vi "map.vi"() -> ()   [LabVIEW 2024]
uses:
  C:/Program Files (x86)/National Instruments/LabVIEW 2024/examples/Design Patterns/Queued Message Handler/support/QMH Fundamentals - Message Cluster.ctl
  <extravilib>/ChannelInstances/Lossy Stream-c(i32)/Read With Abort.vi
  <extravilib>/ChannelInstances/Lossy Stream-c(u16)/Write With Abort.vi
  <extravilib>/ChannelInstances/Lossy Stream-c(u16)/Read With Abort.vi
  <extravilib>/ChannelInstances/Lossy Stream-c(i32)/Write With Abort.vi
  <extravilib>/ChannelInstances/Lossy Stream-c(i32)/EndpointRead.vi
  <extravilib>/ChannelInstances/Lossy Stream-c(u16)/Endpoint.vi
  <extravilib>/ChannelInstances/Lossy Stream-c(u16)/EndpointRead.vi
  <extravilib>/ChannelInstances/Lossy Stream-c(i32)/Endpoint.vi
  ID_List.vi
  isMapRun.vi
  <extravilib>/ChannelInstances/Lossy Stream-c(i32)/Instantiate.vi
  <extravilib>/ChannelInstances/Lossy Stream-c(i32)/)Channel.vi
  <resource>/ChannelSupport/_ChannelSupport/WaitIfNeeded.vi
  <extravilib>/ChannelInstances/Lossy Stream-c(u16)/Instantiate.vi
  <extravilib>/ChannelInstances/Lossy Stream-c(u16)/)Channel.vi
  API_Key.vi
  D:/Autonomous Systems/Oulu/Measurment Systems/EnvironmentalMonitoringSystem/GMapControl/GMapControl/bin/Debug/GMapControl.dll
  GMapControl/GMapControl/bin/Debug/GMapControl.dll
  <extravilib>/ChannelInstances/Lossy Stream-c(u16).lvlib
  <extravilib>/ChannelInstances/Lossy Stream-c(i32).lvlib
  sensor_List.vi
panel:
  out "Range":u16
  out "API_key_delievered":bool=TRUE
  out "GetLastAction":i32
  out "id_list":u16[](array[numeric])
  out "GetLongitude":dbl
  out "GetLatitude":dbl
  out "Button":u16
  out "mouse event":bool
  in  "MapControl":refnum<k24>(container)
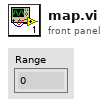
[diagram p1: front panel]
types:
  T1 = typedef "QMH Fundamentals - Message Cluster.ctl" = cluster{"Message":string, "Message Data":variant}
  T2 = typedef "Lossy Stream-c(u16).lvlib/)Channel.ctl" = refnum<queue>
  T3 = typedef "Lossy Stream-c(i32).lvlib/)Channel.ctl" = refnum<queue>
  T4 = cluster{"meta":cluster{"name":string, "website":string, "page":dbl, "limit":dbl}, "results":cluster{"id":i32, "name":string, "distance":dbl, "coordinates":cluster{"latitude":dbl, "longitude":dbl}}[]}
  T5 = cluster{"id":i32, "name":string, "distance":dbl, "coordinates":cluster{"latitude":dbl, "longitude":dbl}}[]
  T6 = cluster{"results":cluster{"id":u16, "latest":cluster{"value":dbl, "datetime":cluster{"utc":string}}, "name":string}[]}
  T7 = cluster{"id":u16, "latest":cluster{"value":dbl, "datetime":cluster{"utc":string}}, "name":string}[]
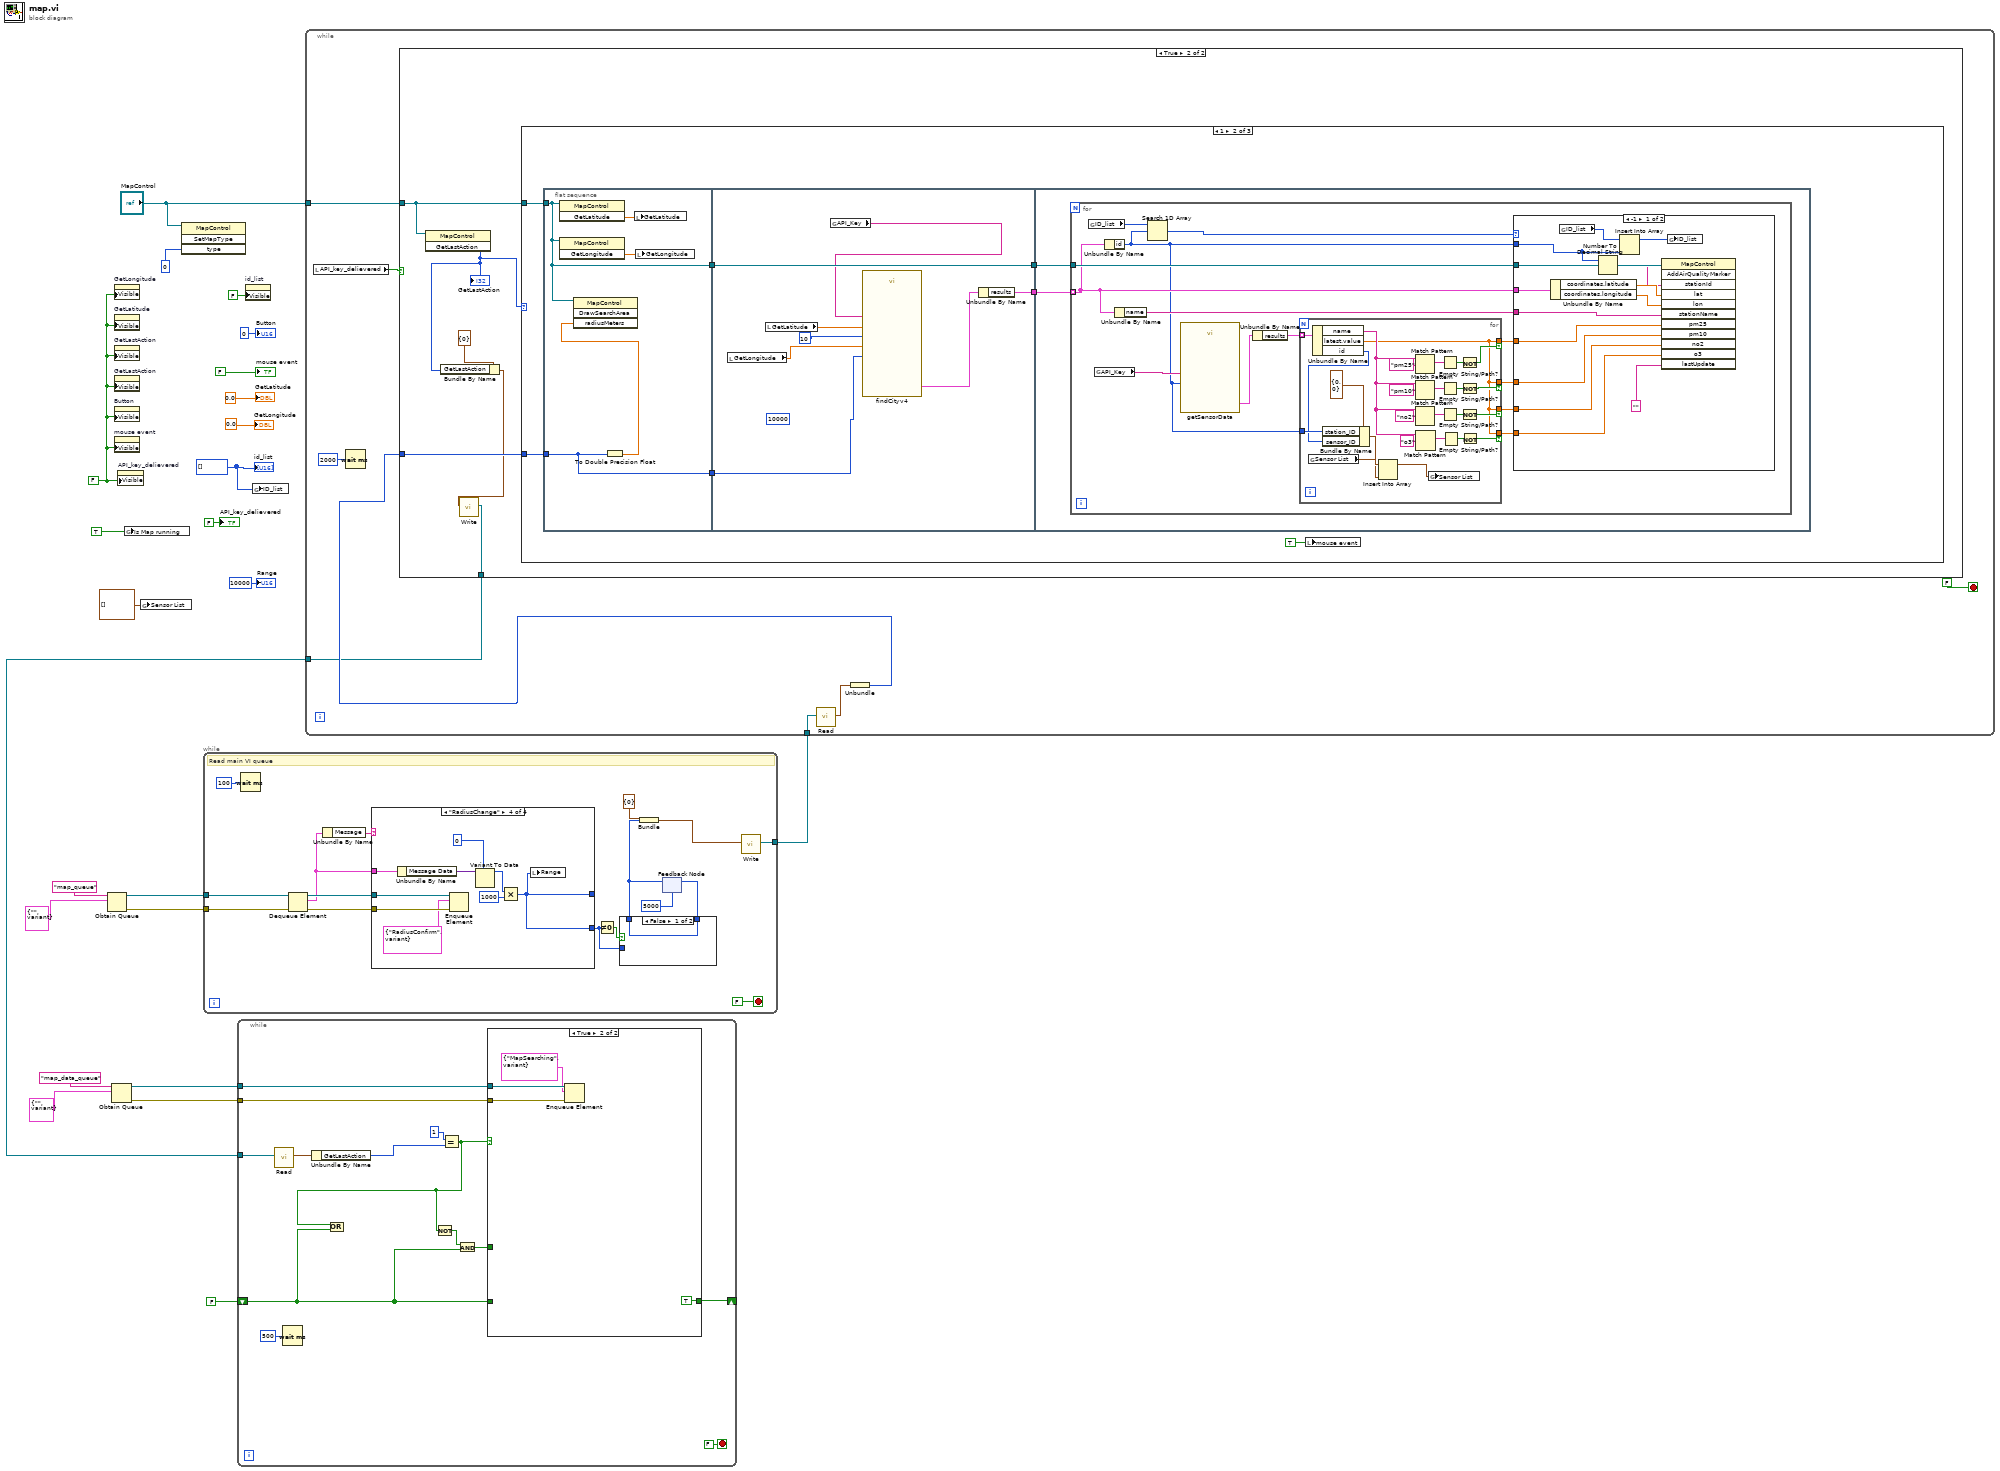
[diagram p0: block diagram]
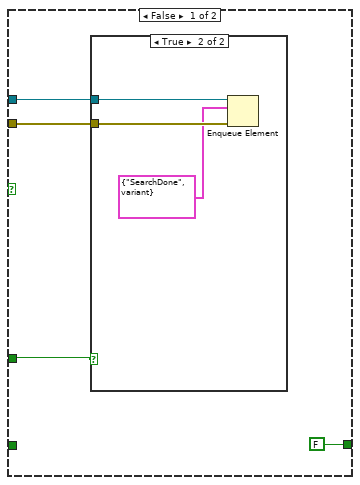
[diagram p2: hidden frame]
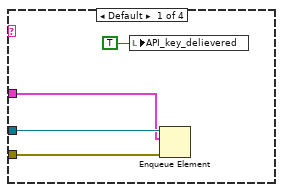
[diagram p5: hidden frame]
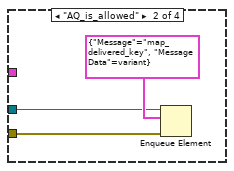
[diagram p6: hidden frame]
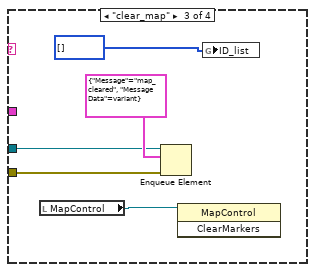
[diagram p7: hidden frame]
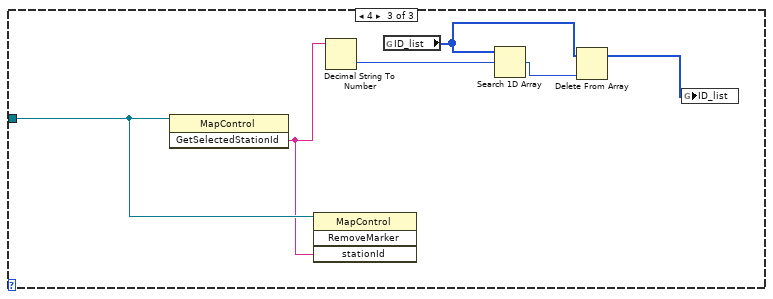
[diagram p11: hidden frame]
diagram:
  w14 = FALSE ("Visible")
  w12 = u16[] [] ("id_list")
  n1 = Obtain Queue(name (unnamed)="map_queue", element data type=T1 {"Message"="", "Message Data"=variant} ("Message Cluster")) -> (queue out=w8:refnum<queue>, error out=w7:errorcluster)  [unwired: 3 in, 1 out]
  n2 = Obtain Queue(name (unnamed)="map_data_queue", element data type=T1 {"Message"="", "Message Data"=variant} ("Message Cluster")) -> (queue out=w3:refnum<queue>, error out=w2:errorcluster)  [unwired: 3 in, 1 out]
  n3 = property on="GetLongitude" class="DigNum (strict)"("Visible"=w14) -> ()  [unwired: 2 in, 2 out]
  n4 = property on="GetLatitude" class="DigNum (strict)"("Visible"=w14) -> ()  [unwired: 2 in, 2 out]
  n5 = property on="GetLastAction" class="DigNum (strict)"("Visible"=w14) -> ()  [unwired: 2 in, 2 out]
  n6 = property on="GetLastAction" class="DigNum (strict)"("Visible"=w14) -> ()  [unwired: 2 in, 2 out]
  n7 = property on="Button" class="DigNum (strict)"("Visible"=w14) -> ()  [unwired: 2 in, 2 out]
  n8 = property on="mouse event" class="Bool (strict)"("Visible"=w14) -> ()  [unwired: 2 in, 2 out]
  n9 = property on="API_key_delievered" class="Bool (strict)"("Visible"=w14) -> ()  [unwired: 2 in, 2 out]
  n10 = global write "isMapRun.vi" "Is Map running"(TRUE ("Is Map running")) -> ()
  n11 = global write "sensor_List.vi" "Sensor List"(cluster{"station_ID":u32, "sensor_ID":u32}[] [] ("Sensor List")) -> ()
  n12 = invoke class="MapControl" method="SetMapType"(reference="MapControl", "type"=0) -> ()  [unwired: 2 in, 4 out]
  n13 = while {
    tunnel: w8 -> [w40]
    tunnel: w7 -> [w39]
    tunnel: [w36] -> w10
    stop <- FALSE stop-if-true
    # "Read main VI queue"
    n14 = Wait (ms)(milliseconds to wait=u32 100) -> ()  [unwired: 1 out]
    n15 = Dequeue Element(queue=w40, error in (no error)=w39) -> (queue out=w33:refnum<queue>, element=w31:T1, error out=w32:errorcluster)  [unwired: 1 in, 1 out]
    n16 = Unbundle By Name(w31) -> ("Message"=w34:string)
    n17 = case shown="\"RadiusChange\"" w34 {
      tunnel: w33 -> [w46 w48 w53 w58]
      tunnel: w32 -> [w45 w47 w52 w57]
      tunnel: w31 -> [w44 _ _ w63]
      tunnel: [_ _ _ w55] -> _
      tunnel: [_ _ _ w55] -> w28
      frame Default {
        n18 = local write "API_key_delievered"(TRUE ("API_key_delievered")) -> ()
        n19 = Enqueue Element(queue=w46, element=w44, error in (no error)=w45) -> ()  [unwired: 1 in, 3 out]
      }
      frame "AQ_is_allowed" {
        n20 = Enqueue Element(queue=w48, element=T1 {"Message"="map_delivered_key", "Message Data"=variant}, error in (no error)=w47) -> ()  [unwired: 1 in, 3 out]
      }
      frame "clear_map" {
        n21 = local read "MapControl"() -> (w51:refnum<k24>)
        n22 = Enqueue Element(queue=w53, element=T1 {"Message"="map_cleared", "Message Data"=variant}, error in (no error)=w52) -> ()  [unwired: 1 in, 3 out]
        n23 = invoke class="MapControl" method="ClearMarkers"(reference=w51) -> ()  [unwired: 2 in, 3 out]
        n24 = global write "ID_List.vi" "ID_list"(u16[] [] ("id_list")) -> ()
      }
      frame "RadiusChange" {
        n25 = Unbundle By Name(w63) -> ("Message Data"=w62:variant)
        n26 = Enqueue Element(queue=w58, element=T1 {"Message"="RadiusConfirm", "Message Data"=variant}, error in (no error)=w57) -> ()  [unwired: 1 in, 3 out]
        n27 = Variant To Data(type=u16 0 ("Numeric"), Variant=w62) -> (data=w60:u16)  [unwired: 1 in, 1 out]
        n28 = Multiply(x=w60, y=u16 1000) -> (x*y=w55:u16)
        n29 = local write "Range"(w55) -> ()
      }
    }
    n30 = Not Equal To 0?(x=w28) -> (x != 0?=w29:bool)
    n31 = feedback #1(u16 5000 ("range")) -> (w26:u16)
    n32 = case shown="False" w29 {
      tunnel: [w41 w42] -> w27
      tunnel: w28 -> [_ w42]
      tunnel: w26 -> [w41 _]
      frame False {
      }
      frame True {
      }
    }
    n33 = Bundle(cluster=cluster{"range":u16} {"range"=0}, "range"=w26) -> (w35:cluster{"range":u16})
    n34 = feedback-in #1(w27) -> ()
    n35 = call <extravilib>:"Write.vi"("element"=w35) -> ("channel"=w36:T2)  [unwired: 8 in, 2 out]
  }
  n36 = property on="id_list" class="Arr (strict)"("Visible"=FALSE) -> ()  [unwired: 2 in, 2 out]
  n37 = global write "ID_List.vi" "ID_list"(w12) -> ()
  n38 = while {
    tunnel: "MapControl" -> [w69]
    tunnel: w10 -> [w67]
    tunnel: [w64] -> w9
    stop <- FALSE stop-if-true
    n39 = local read "API_key_delievered"() -> (w68:bool)
    n40 = Wait (ms)(milliseconds to wait=u32 2000) -> ()  [unwired: 1 out]
    n41 = call <extravilib>:"Read.vi"("channel"=w67) -> ("element"=w66:cluster{"range":u16})  [unwired: 5 in, 5 out]
    n42 = Unbundle(w66) -> ("range"=w65:u16)
    n43 = case shown="True" w68 {
      tunnel: w69 -> [_ w77]
      tunnel: w65 -> [_ w76]
      tunnel: [_ w72] -> w64
      frame False {
      }
      frame True {
        n44 = invoke class="MapControl" method="GetLastAction"(reference=w77) -> ("GetLastAction"=w75:i32)  [unwired: 2 in, 2 out]
        "GetLastAction" <- w75
        n45 = Bundle By Name(cluster=cluster{"GetLastAction":i32} {"GetLastAction"=0} ("input cluster"), "GetLastAction"=w75) -> (w73:cluster{"GetLastAction":i32})
        n46 = call <extravilib>:"Write.vi"("element"=w73) -> ("channel"=w72:T3)  [unwired: 8 in, 2 out]
        n47 = case shown="1" w75 {
          tunnel: w77 -> [_ w84 w157]
          tunnel: w76 -> [_ w78 _]
          frame Default {
          }
          frame 1 {
            n48 = flat-sequence {
              tunnel: [w87] -> w82
              tunnel: [w85] -> w79
              tunnel: w84 -> [w87]
              tunnel: w78 -> [w85]
              tunnel: w82 -> [w97]
              tunnel: [w97] -> w81
              tunnel: [w96] -> w80
              tunnel: w79 -> [w90]
              tunnel: w81 -> [w99]
              tunnel: w80 -> [w98]
              frame #0 {
                n49 = invoke class="MapControl" method="GetLatitude"(reference=w87) -> ("GetLatitude"=w89:dbl)  [unwired: 2 in, 2 out]
                n50 = invoke class="MapControl" method="GetLongitude"(reference=w87) -> ("GetLongitude"=w88:dbl)  [unwired: 2 in, 2 out]
                n51 = To Double Precision Float(number=w85) -> (double precision float=w86:dbl)
                n52 = invoke class="MapControl" method="DrawSearchArea"(reference=w87, "radiusMeters"=w86) -> ()  [unwired: 2 in, 4 out]
                n53 = local write "GetLatitude"(w89) -> ()
                n54 = local write "GetLongitude"(w88) -> ()
              }
              frame #1 {
                (unwired) u16 10000 ("range")
                n55 = local read "GetLongitude"() -> (w93:dbl)
                n56 = local read "GetLatitude"() -> (w95:dbl)
                n57 = global read "API_Key.vi" "API_Key"() -> (w91:string)
                n58 = call "findCityv4.vi"("limit"=u16 10, "API-key"=w91, "longitude"=w93, "latitude"=w95, "range"=w90) -> ("value"=w92:T4)  [unwired: 2 out]
                n59 = Unbundle By Name(w92) -> ("results"=w96:T5)
              }
              frame #2 {
                n60 = for {
                  tunnel: w99 -> [w112]
                  tunnel: w98 -> [w109] mode=indexing
                  n61 = global read "ID_List.vi" "ID_list"() -> (w110:u16[])
                  n62 = global read "API_Key.vi" "API_Key"() -> (w107:string)
                  n63 = Unbundle By Name(w109) -> ("id"=w100:i32)
                  n64 = Unbundle By Name(w109) -> ("name"=w108:string)
                  n65 = Search 1D Array(1D array=w110, element=w100) -> (index of element=w111:i32)  [unwired: 1 in]
                  n66 = call "getSensorData.vi"("API-key"=w107, "station id"=w100) -> ("value"=w106:T6)  [unwired: 3 in, 1 out]
                  n67 = Unbundle By Name(w106) -> ("results"=w105:T7)
                  n68 = for {
                    tunnel: w105 -> [w137] mode=indexing
                    tunnel: [w120] -> w104 if=w133
                    tunnel: [w120] -> w103 if=w126
                    tunnel: [w120] -> w102 if=w125
                    tunnel: [w120] -> w101 if=w119
                    tunnel: w100 -> [w115]
                    n69 = global read "sensor_List.vi" "Sensor List"() -> (w118:cluster{"station_ID":u32, "sensor_ID":u32}[])
                    n70 = Unbundle By Name(w137) -> ("name"=w121:string, "latest.value"=w120:dbl, "id"=w113:u16)
                    n71 = Bundle By Name(cluster=cluster{"station_ID":i32, "sensor_ID":i32} {"station_ID"=0, "sensor_ID"=0}, "station_ID"=w115, "sensor_ID"=w113) -> (w114:cluster{"station_ID":i32, "sensor_ID":i32})
                    n72 = Insert Into Array(array=w118, new element=w114) -> (w117:cluster{"station_ID":u32, "sensor_ID":u32}[])  [unwired: 1 in]
                    n73 = Match Pattern(string=w121, regular expression="pm25") -> (match substring=w135:string)  [unwired: 1 in, 3 out]
                    n74 = Match Pattern(string=w121, regular expression="pm10") -> (match substring=w131:string)  [unwired: 1 in, 3 out]
                    n75 = Match Pattern(string=w121, regular expression="no2") -> (match substring=w128:string)  [unwired: 1 in, 3 out]
                    n76 = Match Pattern(string=w121, regular expression="o3") -> (match substring=w123:string)  [unwired: 1 in, 3 out]
                    n77 = global write "sensor_List.vi" "Sensor List"(w117) -> ()
                    n78 = Empty String/Path?(string/path=w135) -> (empty?=w134:bool)
                    n79 = Empty String/Path?(string/path=w131) -> (empty?=w130:bool)
                    n80 = Empty String/Path?(string/path=w128) -> (empty?=w127:bool)
                    n81 = Empty String/Path?(string/path=w123) -> (empty?=w122:bool)
                    n82 = Not(x=w134) -> (.not. x?=w133:bool)
                    n83 = Not(x=w130) -> (.not. x?=w126:bool)
                    n84 = Not(x=w127) -> (.not. x?=w125:bool)
                    n85 = Not(x=w122) -> (.not. x?=w119:bool)
                  }
                  n86 = case shown="-1" w111 {
                    tunnel: w112 -> [w151 _]
                    tunnel: w109 -> [w150 _]
                    tunnel: w100 -> [w146 _]
                    tunnel: w108 -> [w142 _]
                    tunnel: w104 -> [w141 _]
                    tunnel: w103 -> [w140 _]
                    tunnel: w102 -> [w139 _]
                    tunnel: w101 -> [w138 _]
                    frame -1 {
                      n87 = Unbundle By Name(w150) -> ("coordinates.latitude"=w147:dbl, "coordinates.longitude"=w148:dbl)
                      n88 = global read "ID_List.vi" "ID_list"() -> (w144:u16[])
                      n89 = Number To Decimal String(number=w146) -> (decimal integer string=w145:string)  [unwired: 1 in]
                      n90 = Insert Into Array(array=w144, new element=w146) -> (w143:u16[])  [unwired: 1 in]
                      n91 = invoke class="MapControl" method="AddAirQualityMarker"(reference=w151, "stationId"=w145, "lat"=w147, "lon"=w148, "stationName"=w142, "pm25"=w141, "pm10"=w140, "no2"=w139, "o3"=w138, "lastUpdate"="") -> ()  [unwired: 2 in, 12 out]
                      n92 = global write "ID_List.vi" "ID_list"(w143) -> ()
                    }
                    frame Default {
                    }
                  }
                }
              }
            }
            n93 = local write "mouse event"(TRUE ("mouse event")) -> ()
          }
          frame 4 {
            n94 = invoke class="MapControl" method="GetSelectedStationId"(reference=w157) -> ("GetSelectedStationId"=w156:string)  [unwired: 2 in, 2 out]
            n95 = invoke class="MapControl" method="RemoveMarker"(reference=w157, "stationId"=w156) -> ()  [unwired: 2 in, 4 out]
            n96 = Decimal String To Number(string=w156) -> (number=w155:i32)  [unwired: 2 in, 1 out]
            n97 = global read "ID_List.vi" "ID_list"() -> (w152:u16[])
            n98 = Search 1D Array(1D array=w152, element=w155) -> (index of element=w154:i32)  [unwired: 1 in]
            n99 = Delete From Array(array=w152, index=w154) -> (array with subset deleted=w153:u16[])  [unwired: 1 in, 1 out]
            n100 = global write "ID_List.vi" "ID_list"(w153) -> ()
          }
        }
      }
    }
  }
  n101 = while {
    tunnel: w9 -> [w167]
    tunnel: w3 -> [w166]
    tunnel: w2 -> [w165]
    shift-right: [w160] -> _
    shift-left: FALSE -> [w158]
    stop <- FALSE stop-if-true
    n102 = call <extravilib>:"Read.vi"("channel"=w167) -> ("element"=w169:cluster{"GetLastAction":i32})  [unwired: 5 in, 5 out]
    n103 = Wait (ms)(milliseconds to wait=u32 500) -> ()  [unwired: 1 out]
    n104 = Unbundle By Name(w169) -> ("GetLastAction"=w163:i32)
    n105 = Equal?(x=1, y=w163) -> (x = y?=w159:bool)
    n106 = Or(x=w159, y=w158) -> ()  [unwired: 1 out]
    n107 = Not(x=w159) -> (.not. x?=w162:bool)
    n108 = And(x=w162, y=w158) -> (x .and. y?=w161:bool)
    n109 = case shown="True" w159 {
      tunnel: w166 -> [w173 w181]
      tunnel: w165 -> [w172 w180]
      tunnel: w161 -> [w174 _]
      tunnel: w158 -> [_ _]
      tunnel: [FALSE TRUE] -> w160
      frame False {
        n110 = case shown="True" w174 {
          tunnel: w173 -> [_ w177]
          tunnel: w172 -> [_ w176]
          frame False {
          }
          frame True {
            n111 = Enqueue Element(queue=w177, element=T1 {"Message"="SearchDone", "Message Data"=variant}, error in (no error)=w176) -> ()  [unwired: 1 in, 3 out]
          }
        }
      }
      frame True {
        n112 = Enqueue Element(queue=w181, element=T1 {"Message"="MapSearching", "Message Data"=variant}, error in (no error)=w180) -> ()  [unwired: 1 in, 3 out]
      }
    }
  }
  "mouse event" <- FALSE ("mouse event")
  "Button" <- u16 0 ("Button")
  "GetLatitude" <- 0.0 ("GetLatitude")
  "GetLongitude" <- 0.0 ("GetLongitude")
  "id_list" <- w12
  "API_key_delievered" <- FALSE ("Boolean")
  "Range" <- u16 10000 ("Numeric")
